vi "destroyEvents.vi"(8 "error in (no error)":errorcluster, 11 "SAL_Events in":refnum<class "SAL_Events.lvclass">) -> (0 "error out":errorcluster, 3 "SAL_Events out":refnum<class "SAL_Events.lvclass">)   [LabVIEW 2015, in "SAL_Events.lvclass"]
uses:
  SAL_Events.lvclass
  SAL_Events.lvclass/SAL_Events.ctl
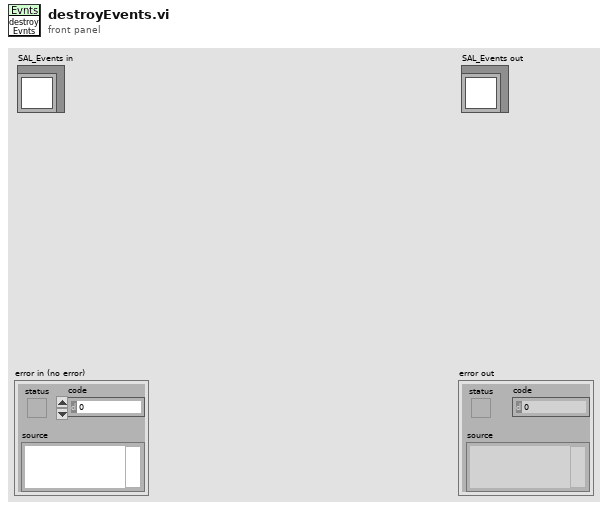
[diagram p1: front panel]
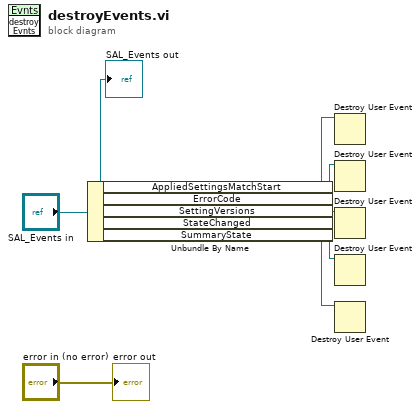
[diagram p0: block diagram]
diagram:
  n1 = Unbundle By Name("SAL_Events in") -> ("AppliedSettingsMatchStart"=w5:refnum<user-event>, "ErrorCode"=w4:refnum<user-event>, "SettingVersions"=w3:refnum<user-event>, "StateChanged"=w2:refnum<user-event>, "SummaryState"=w1:refnum<user-event>)
  n2 = Destroy User Event(user event=w5) -> ()  [unwired: 1 in, 1 out]
  n3 = Destroy User Event(user event=w4) -> ()  [unwired: 1 in, 1 out]
  n4 = Destroy User Event(user event=w3) -> ()  [unwired: 1 in, 1 out]
  n5 = Destroy User Event(user event=w2) -> ()  [unwired: 1 in, 1 out]
  n6 = Destroy User Event(user event=w1) -> ()  [unwired: 1 in, 1 out]
  "error out" <- "error in (no error)"
  "SAL_Events out" <- "SAL_Events in"
